vi "gui-camera-disabled-array.vi"(0 "general-camera-status":T1) -> (1 "enabled detectors":i32[](array[numeric]), 2 "disabled detectors":i32[](array[numeric]))   [LabVIEW 2015]
panel:
  # "Init"
  # "Cooling"
  # "Parameters"
  # "Newton"
  # "iDus"
  # "Clara"
  # "Xeva"
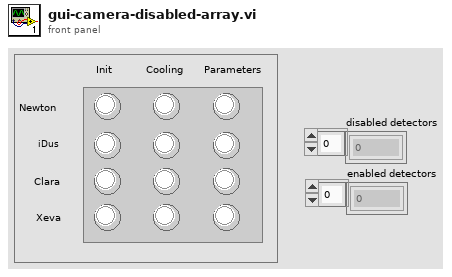
[diagram p1: front panel]
types:
  T1 = cluster{"Newton Init":bool, "Newton Cooling":bool, "Newton Parameters ":bool, "iDus Init":bool, "iDus Cooling":bool, "iDus Parameters":bool, "Clara Init":bool, "Clara Cooling":bool, "Clara Parameters":bool, "Xeva-init":bool, "xeva-cooling":bool, "xeva-parameters":bool}
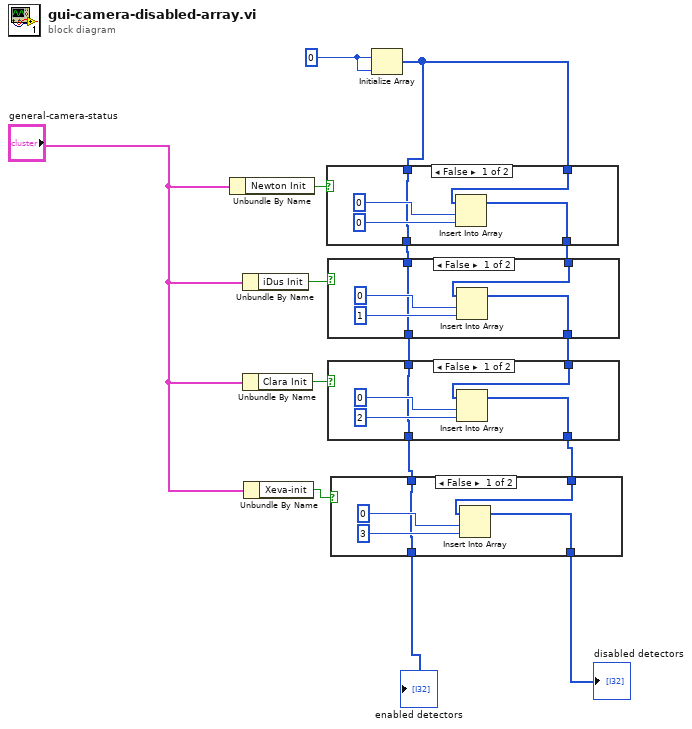
[diagram p0: block diagram]
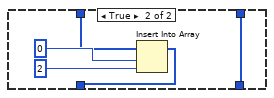
[diagram p2: hidden frame]
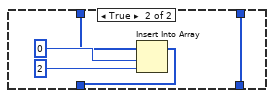
[diagram p3: hidden frame]
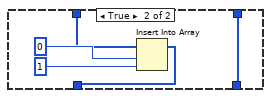
[diagram p4: hidden frame]
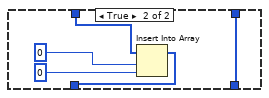
[diagram p5: hidden frame]
diagram:
  w15 = 0
  n1 = Unbundle By Name("general-camera-status") -> ("Newton Init"=w14:bool)
  n2 = Unbundle By Name("general-camera-status") -> ("iDus Init"=w13:bool)
  n3 = Unbundle By Name("general-camera-status") -> ("Clara Init"=w11:bool)
  n4 = Unbundle By Name("general-camera-status") -> ("Xeva-init"=w2:bool)
  n5 = Initialize Array(w15, w15) -> (w9:i32[])
  n6 = case shown="False" w14 {
    tunnel: [w18 w25] -> w10
    tunnel: w9 -> [w17 w25]
    tunnel: w9 -> [w16 w22]
    tunnel: [w16 w21] -> w8
    frame False {
      n7 = Insert Into Array(array=w17, index=0, new element=0 ("new element/subarray")) -> (w18:i32[])
    }
    frame True {
      n8 = Insert Into Array(array=w22, index=0, new element=0 ("new element/subarray")) -> (w21:i32[])
    }
  }
  n9 = case shown="False" w13 {
    tunnel: [w28 w35] -> w12
    tunnel: w10 -> [w27 w35]
    tunnel: w8 -> [w26 w32]
    tunnel: [w26 w31] -> w7
    frame False {
      n10 = Insert Into Array(array=w27, index=0, new element=1 ("new element/subarray")) -> (w28:i32[])
    }
    frame True {
      n11 = Insert Into Array(array=w32, index=0, new element=1 ("new element/subarray")) -> (w31:i32[])
    }
  }
  n12 = case shown="False" w11 {
    tunnel: [w38 w45] -> w4
    tunnel: w12 -> [w37 w45]
    tunnel: w7 -> [w36 w42]
    tunnel: [w36 w41] -> w6
    frame False {
      n13 = Insert Into Array(array=w37, index=0, new element=2 ("new element/subarray")) -> (w38:i32[])
    }
    frame True {
      n14 = Insert Into Array(array=w42, index=0, new element=2 ("new element/subarray")) -> (w41:i32[])
    }
  }
  n15 = case shown="False" w2 {
    tunnel: [w48 w55] -> w3
    tunnel: w4 -> [w47 w55]
    tunnel: w6 -> [w46 w52]
    tunnel: [w46 w51] -> w5
    frame False {
      n16 = Insert Into Array(array=w47, index=0, new element=3 ("new element/subarray")) -> (w48:i32[])
    }
    frame True {
      n17 = Insert Into Array(array=w52, index=0, new element=2 ("new element/subarray")) -> (w51:i32[])
    }
  }
  "disabled detectors" <- w3
  "enabled detectors" <- w5
